vi "Get or Create Folder.vi"(8 "error in (no error)":errorcluster, 9 "CreateAsProperties":bool, 10 "Virtual Folder Name":string, 11 "BaseAccessorScripter in":refnum<class "BaseAccessorScripter.lvclass">) -> (0 "error out":errorcluster, 2 "Folder Refnum out":refnum<vi>, 3 "BaseAccessorScripter out":refnum<class "BaseAccessorScripter.lvclass">)   [LabVIEW 2021, in "MemberVICreation.lvlib" / "BaseAccessorScripter.lvclass"]
uses:
  <resource>/Framework/Providers/LVClassLibrary/NewAccessors/BaseAccessorScripter/BaseAccessorScripter.lvclass
  <resource>/Framework/Providers/LVClassLibrary/NewAccessors/BaseAccessorScripter/BaseAccessorScripter.lvclass/BaseAccessorScripter.ctl
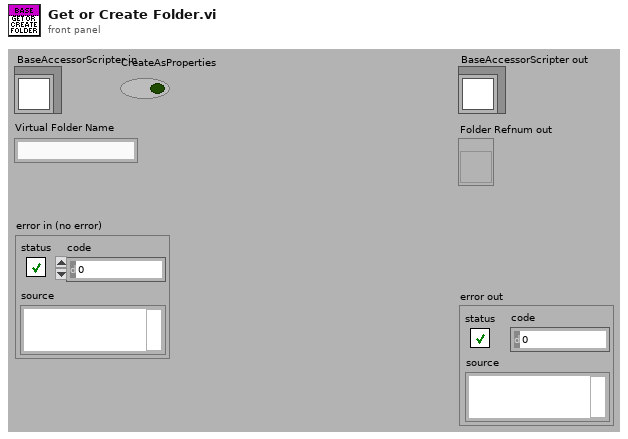
[diagram p1: front panel]
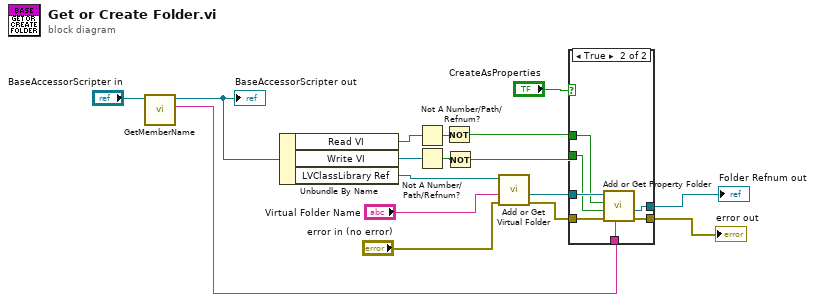
[diagram p0: block diagram]
diagram:
  n1 = call-dynamic "GetMemberName.vi"("BaseAccessorScripter in"="BaseAccessorScripter in") -> ("MemberName"=w9:string, "BaseAccessorScripter out"=w3:refnum<class "BaseAccessorScripter.lvclass">)  [unwired: 1 in, 8 out]
  "BaseAccessorScripter out" <- w3
  n2 = Unbundle By Name(w3) -> ("Read VI"=w2:refnum<vi>, "Write VI"=w1:refnum<vi>, "LVClassLibrary Ref"=w8:refnum<vi>)
  n3 = Not A Number/Path/Refnum?(number/path/refnum=w2) -> (NaN/Path/Refnum?=w7:bool)
  n4 = Not A Number/Path/Refnum?(number/path/refnum=w1) -> (NaN/Path/Refnum?=w6:bool)
  n5 = Not(x=w7) -> (.not. x?=w5:bool)
  n6 = Not(x=w6) -> (.not. x?=w4:bool)
  n7 = call <resource>:"Add or Get Virtual Folder.vi"("error in (no error)"="error in (no error)", "Virtual Folder Name"="Virtual Folder Name", "LVClassLibrary Refnum in"=w8) -> ("error out"=w16:errorcluster, "Folder Refnum out"=w15:refnum<vi>)  [unwired: 6 in, 1 out]
  n8 = case shown="True" "CreateAsProperties" {
    tunnel: w15 -> [w19 w23]
    tunnel: w16 -> [w18 w26]
    tunnel: [w19 w24] -> w13
    tunnel: [w18 w25] -> w12
    tunnel: w9 -> [_ w22]
    tunnel: w5 -> [_ w21]
    tunnel: w4 -> [_ w20]
    frame False {
    }
    frame True {
      n9 = call <resource>:"Add or Get Property Folder.vi"("Property Folder Name"=w22, "error in (no error)"=w26, "WantsWrite"=w20, "WantsRead"=w21, "Parent ProjectItem Refnum in"=w23) -> ("error out"=w25:errorcluster, "Folder Refnum out"=w24:refnum<vi>)  [unwired: 4 in, 1 out]
    }
  }
  "Folder Refnum out" <- w13
  "error out" <- w12
